vi "Actor Teardown.vi"(10 "Error":errorcluster, 11 "Process in":refnum<class "ABD.lvclass">) -> (0 "error out":errorcluster, 2 "Teardown?":bool, 3 "Process out":refnum<class "ABD.lvclass">)   [LabVIEW 2021, in "ABD.lvlib" / "ABD.lvclass"]
uses:
  ABD.lvclass
  ABD.lvclass/ABD.ctl
  LVCAM/LVCAM/Actor/Actor.lvclass
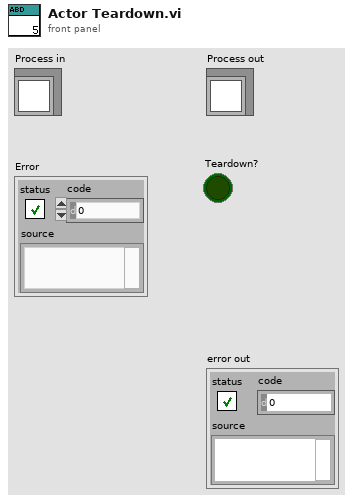
[diagram p1: front panel]
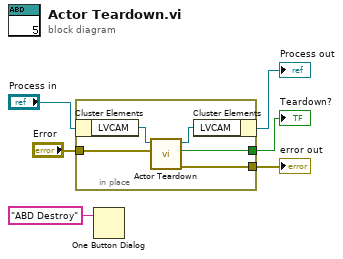
[diagram p0: block diagram]
diagram:
  n1 = in-place {
    in-place-border: "Error" -> [w11]
    in-place-border: [w10] -> w4
    in-place-border: [w9] -> w3
    n2 = in-place-cluster #1("Process in") -> ("LVCAM"=w8:refnum<class "Actor.lvclass">)
    n3 = call-dynamic "Actor Teardown.vi"("Error"=w11, "Actor in"=w8) -> ("error out"=w10:errorcluster, "Teardown?"=w9:bool, "Actor out"=w7:refnum<class "Actor.lvclass">)  [unwired: 7 in]
    n4 = in-place-cluster #1("LVCAM"=w7) -> (→"Process out":refnum<class "ABD.lvclass">)
  }
  "Teardown?" <- w3
  "error out" <- w4
  n5 = One Button Dialog(message="ABD Destroy") -> ()  [unwired: 1 in, 1 out]
